vi "Pressure Box Cali.vi"(8 "Error In":errorcluster) -> (0 "Error Out":errorcluster)   [LabVIEW 2017, in "AnalysisSupport.lvlib"]
uses:
  AnalysisSupport.lvlib
  <vilib>/measure/madcrms.llb/Basic Averaged DC-RMS for 1 Chan.vi
  CollectionSupport.lvlib
  <vilib>/Analysis/NI_AALBase.lvlib
  <vilib>/measure/NI_MAPro.lvlib
panel:
  in  "Add Button HS":bool
  in  "Stop Button HS":bool
  out "Pressure Slope":dbl
  out "Pressure Intercept":dbl
  in  "Pressure Reference":dbl
  out "Pressure DC Voltage":dbl
  out "Pressure Curve":cluster{"Y":dbl[], "Y":dbl[]}[](graph)
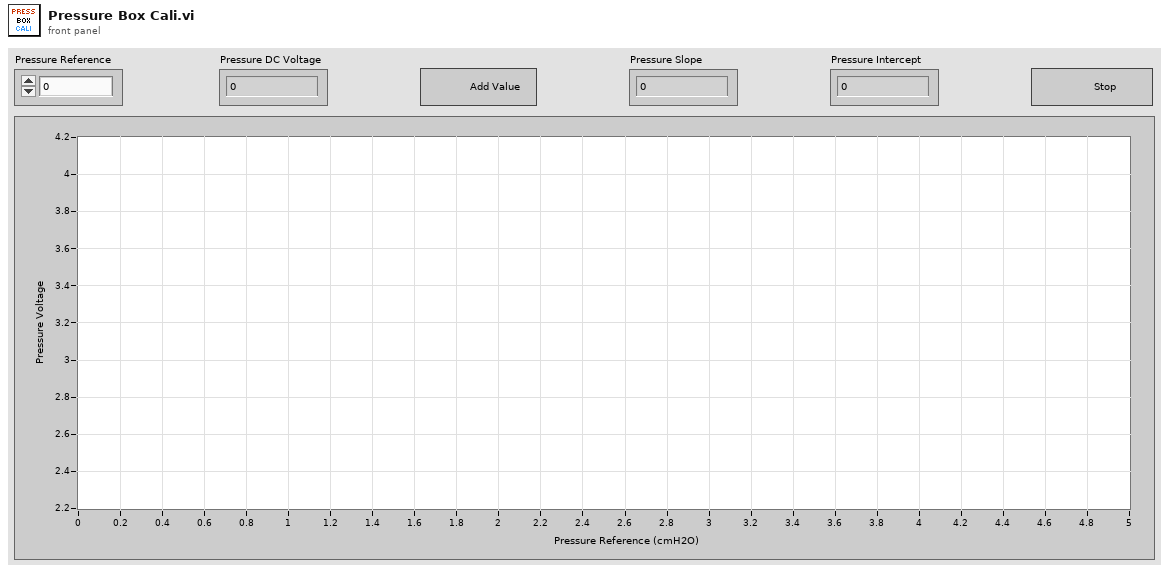
[diagram p1: front panel]
types:
  T1 = enum16{"open", "replace", "create", "open or create", "replace or create", "replace or create with confirmation"}
  T2 = enum8{"Enabled", "Disabled", "Disabled and Grayed Out"}
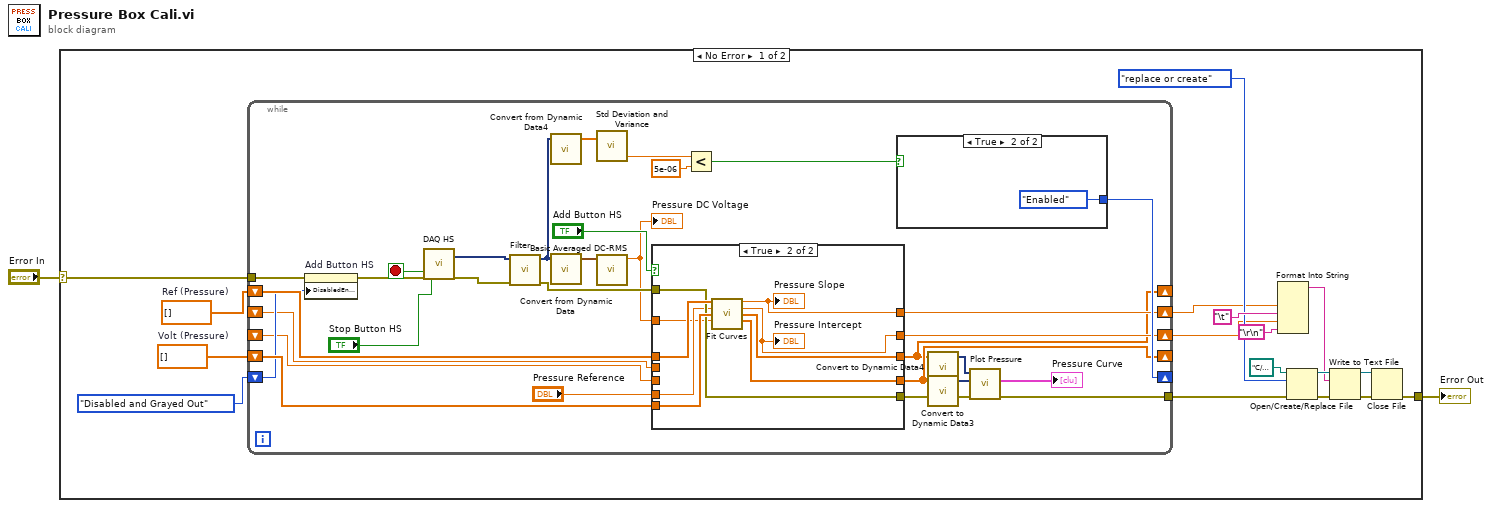
[diagram p0: block diagram]
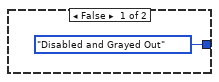
[diagram p2: hidden frame]
diagram:
  n1 = case shown="No Error" "Error In" {
    selector: "Error In" -> [w19 w67]
    tunnel: [w3 w67] -> w1
    frame No Error {
      w17 = dbl[] []  # Ref (Pressure)
      w18 = dbl[] []  # Volt (Pressure)
      n2 = while {
        tunnel: w19 -> [w39]
        shift-right: [w24] -> _
        shift-left: w18 -> [w44]
        shift-right: [w23] -> _
        shift-left: w17 -> [w45]
        shift-right: [w36] -> _
        shift-left: T2."Disabled and Grayed Out" ("Disabled") -> [w37]
        shift-right: [w32] -> w6
        shift-left: _ -> [w30]
        shift-right: [w31] -> w7
        shift-left: _ -> [w29]
        tunnel: [w25] -> w4
        stop <- w46 stop-if-true
        n3 = property on="Add Button HS" class="Bool"(error in=w39, "DisabledEnum"=w37) -> (error out=w38:errorcluster)  [unwired: 1 in, 1 out]
        n4 = call "DAQ HS"("error in"=w38, "stop (F)"="Stop Button HS") -> ("data"=w49:dynamicdata, "stopped"=w46:bool, "error out"=w50:errorcluster)  [unwired: 14 in, 1 out]
        n5 = call "Filter"("error in (no error)"=w50, "Signal"=w49) -> ("error out"=w27:errorcluster, "Filtered Signal"=w22:dynamicdata)  [unwired: 8 in]
        n6 = call "Convert from Dynamic Data4"("Dynamic Data Type"=w22) -> ("Array"=w34:dbl[])  [unwired: 3 in]
        n7 = call "Convert from Dynamic Data"("Dynamic Data Type"=w22) -> ("Waveform"=w21:waveform(dbl))  [unwired: 3 in]
        n8 = call <vilib>:"Std Deviation and Variance.vi"("X"=w34) -> ("variance"=w33:dbl)  [unwired: 1 in, 2 out]
        n9 = call-poly <vilib>:"Basic Averaged DC-RMS.vi"("signal in"=w21) -> ("DC value"=w20:dbl)  [unwired: 7 in, 3 out]
        "Pressure DC Voltage" <- w20
        n10 = case shown="True" "Add Button HS" {
          tunnel: "Pressure Reference" -> [_ w59]
          tunnel: w44 -> [w56 w61]
          tunnel: w45 -> [w57 w62]
          tunnel: w20 -> [_ w58]
          tunnel: [w57 w64] -> w23
          tunnel: [w56 w63] -> w24
          tunnel: [w55 w66] -> w32
          tunnel: [w54 w65] -> w31
          tunnel: w30 -> [w55 _]
          tunnel: w29 -> [w54 _]
          tunnel: w27 -> [w53 w60]
          tunnel: [w53 w60] -> w26
          frame False {
          }
          frame True {
            n11 = call "Fit Curves.vi"("Reference (Array)"=w62, "Reference (Value)"=w59, "Voltage (Array)"=w61, "Voltage (Value)"=w58) -> ("Slope"=w66:dbl, "Intercept"=w65:dbl, "Reference Out"=w64:dbl[], "Voltage Out"=w63:dbl[])  [unwired: 7 in, 1 out]
            "Pressure Slope" <- w66
            "Pressure Intercept" <- w65
          }
        }
        n12 = Less?(x=w33, y=5e-06) -> (x < y?=w28:bool)
        n13 = case shown="True" w28 {
          tunnel: [T2."Disabled and Grayed Out" ("Disabled") T2."Enabled" ("Disabled")] -> w36
          frame False {
          }
          frame True {
          }
        }
        n14 = call "Convert to Dynamic Data4"("Array"=w23) -> ("Dynamic Data Type"=w43:dynamicdata)  [unwired: 3 in]
        n15 = call "Convert to Dynamic Data3"("Array"=w24) -> ("Dynamic Data Type"=w42:dynamicdata)  [unwired: 3 in]
        n16 = call "Plot Pressure"("error in (no error)"=w26, "Y Input"=w42, "X Input"=w43) -> ("error out"=w25:errorcluster, "XY Graph"=→"Pressure Curve":cluster{"Y":dbl[], "Y":dbl[]}[])  [unwired: 7 in]
      }
      n17 = Format Into String(w6, "\t", w7, "\r\n") -> (resulting string=w11:string)  [unwired: 3 in, 1 out]
      n18 = Open/Create/Replace File(file path (use dialog)=path "C:/Users/scholp/Desktop/Calibration .txt files/SH Pressure Cali.txt", error in=w4, operation (0:open)=T1."replace or create") -> (refnum out=w13:refnum<file>, error out=w14:errorcluster)  [unwired: 3 in, 1 out]
      n19 = Write to Text File(file (use dialog)=w13, text=w11, error in=w14) -> (refnum out=w12:refnum<file>, error out=w15:errorcluster)  [unwired: 1 in, 1 out]
      n20 = Close File(refnum=w12, error in=w15) -> (error out=w3:errorcluster)  [unwired: 1 out]
    }
    frame Error {
    }
  }
  "Error Out" <- w1
